vi "Execute.vi"(8 "error in (no error)":errorcluster, 9 "Workspace":T1, 10 "Control In":T2={"I-O.lvclass"=refnum, "Motion.lvclass"=refnum, "Dispenser.lvclass"=refnum}, 11 "Secure Syringe in":refnum<class "SecureRelease Syringe.lvclass">) -> (0 "error out":errorcluster, 2 "Control Out":T2, 3 "Secure Syringe out":refnum<class "SecureRelease Syringe.lvclass">)   [LabVIEW 2016, in "SecureRelease Syringe.lvclass"]
uses:
  SecureRelease Syringe.lvclass
  Controller/Controllers.ctl
  Controller/I-O/I-O.lvclass
  Controller/Motion/A3200/A3200.lvclass
  Controller/Dispenser/Dispenser.lvclass
  Controller/Motion/Motion.lvclass
  Workspace/Workspace.ctl
  SecureRelease Syringe.lvclass/SecureRelease Syringe.ctl
  Dispense/Dispense.lvclass
  Controller/Controller.lvclass
  Workspace/Fixture.lvclass
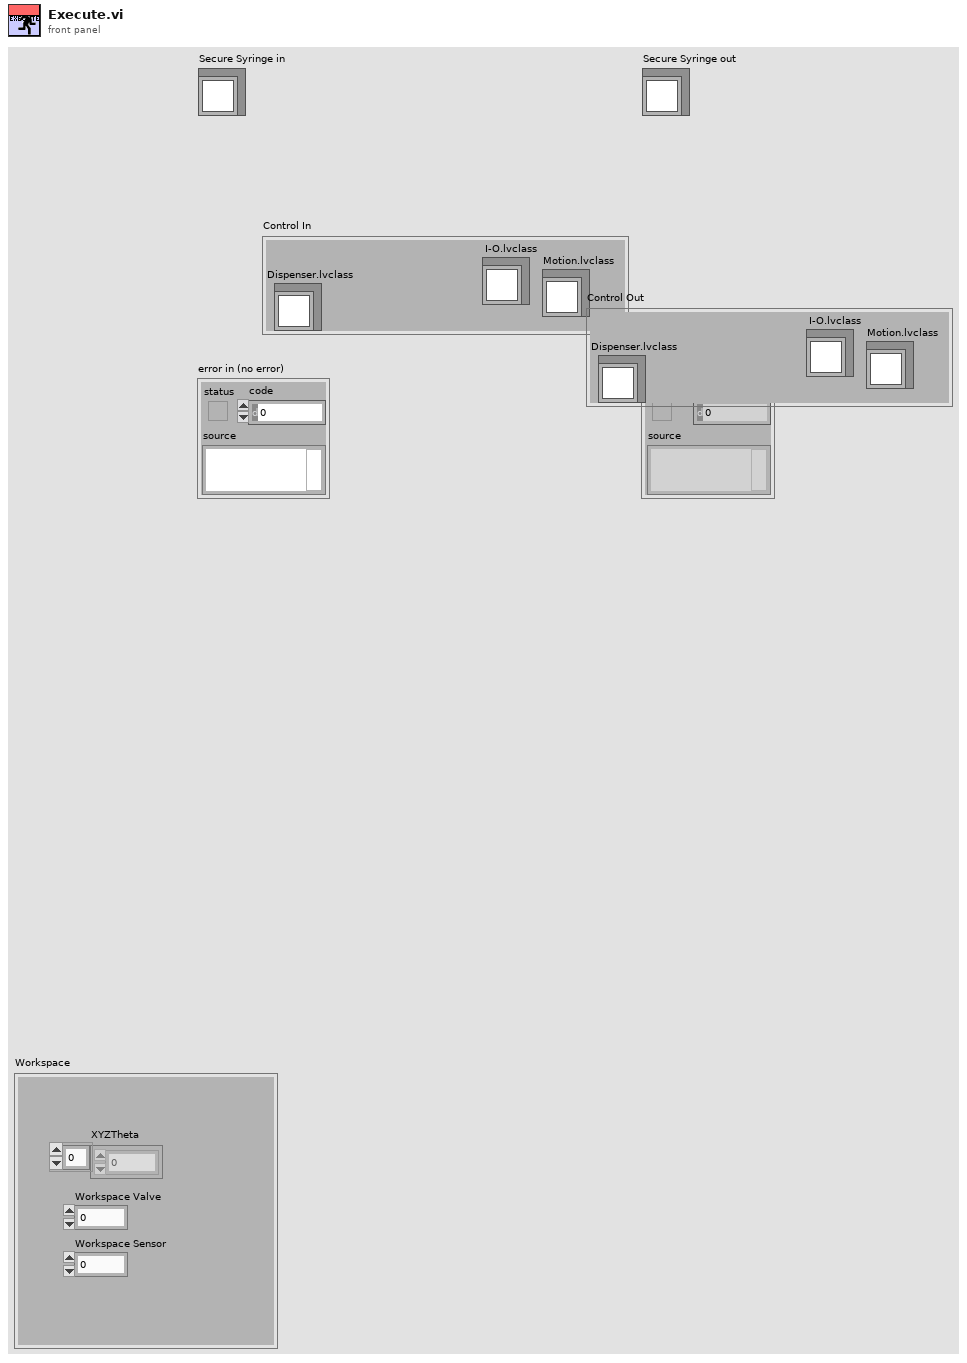
[diagram p1: front panel]
types:
  T1 = typedef "Fixture.lvclass/Workspace.ctl" = cluster{"XYZTheta":dbl[], "Workspace Valve":i32, "Workspace Sensor":i32}
  T2 = typedef "Controller.lvclass/Controllers.ctl" = cluster{"I-O.lvclass":refnum<class "I-O.lvclass">, "Motion.lvclass":refnum<class "Motion.lvclass">, "Dispenser.lvclass":refnum<class "Dispenser.lvclass">}
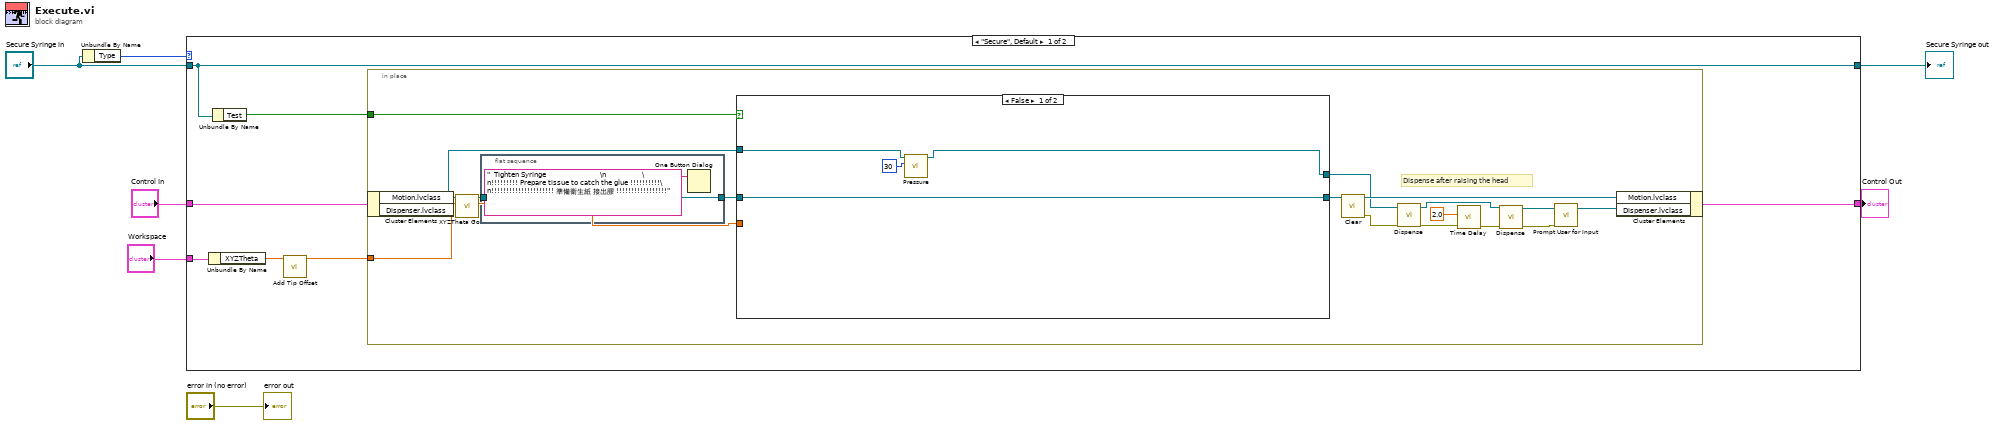
[diagram p0: block diagram]
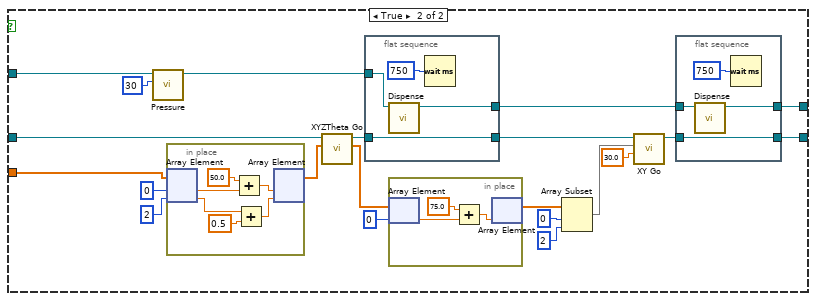
[diagram p2: hidden frame]
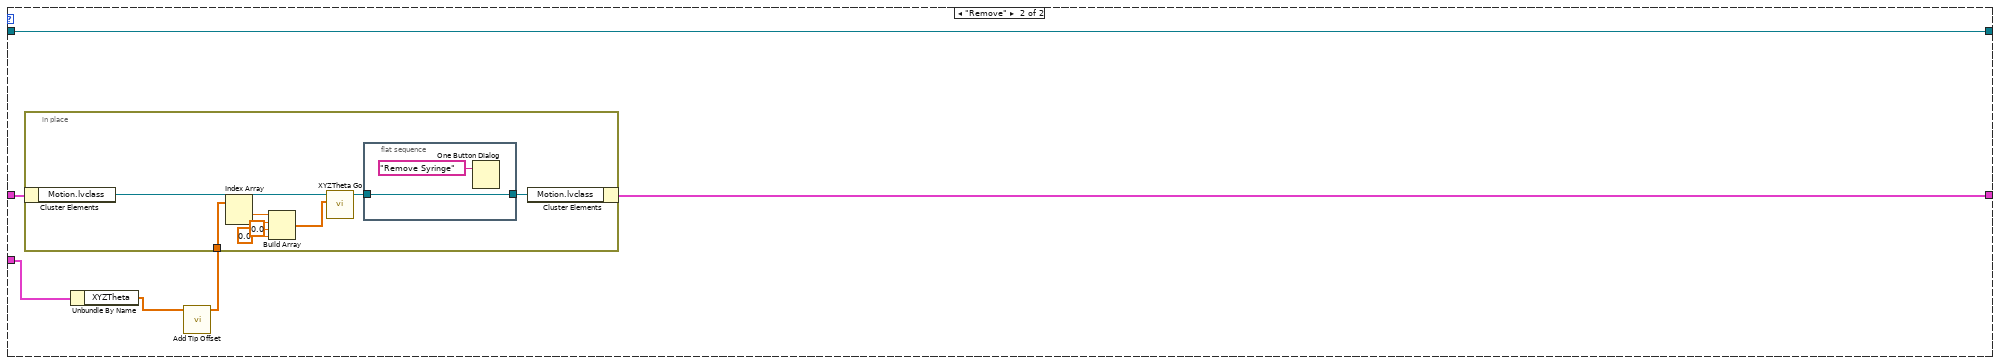
[diagram p3: hidden frame]
diagram:
  n1 = Unbundle By Name("Secure Syringe in") -> ("Type"=w1:enum16{"Secure", "Remove"})
  n2 = case shown="\"Secure\", Default" w1 {
    tunnel: "Workspace" -> [w14 w78]
    tunnel: "Secure Syringe in" -> [w10 w79]
    tunnel: [w10 w79] -> w5
    tunnel: "Control In" -> [w13 w80]
    tunnel: [w12 w81] -> w3
    frame "Secure", Default {
      n3 = Unbundle By Name(w14) -> ("XYZTheta"=w9:dbl[])
      n4 = Unbundle By Name(w10) -> ("Test"=w11:bool)
      n5 = call "Add Tip Offset.vi"("XYZTheta"=w9) -> ("XYZTheta"=w8:dbl[])  [unwired: 10 in]
      n6 = in-place {
        in-place-border: w8 -> [w30]
        in-place-border: w11 -> [w24]
        # "Dispense after raising the head"
        n7 = in-place-cluster #1(w13) -> ("Motion.lvclass"=w31:refnum<class "Motion.lvclass">, "Dispenser.lvclass"=w23:refnum<class "Dispenser.lvclass">)
        n8 = call "XYZTheta Go.vi"("XYZTheta In"=w30, "Motion in"=w31) -> ("XYZTheta Out"=w25:dbl[], "Motion out"=w29:refnum<class "Motion.lvclass">)  [unwired: 7 in, 1 out]
        n9 = flat-sequence {
          tunnel: [w32] -> w27
          tunnel: w29 -> [w32]
          frame #0 {
            n10 = One Button Dialog(message="  Tighten Syringe                           \n                  \n!!!!!!!!! Prepare tissue to catch the glue !!!!!!!!!!\n!!!!!!!!!!!!!!!!!!!!! 準備衛生紙 接出膠 !!!!!!!!!!!!!!!!!") -> ()  [unwired: 1 in, 1 out]
          }
        }
        n11 = case shown="False" w24 {
          tunnel: w27 -> [w37 w58]
          tunnel: [w37 w44] -> w26
          tunnel: w25 -> [_ w57]
          tunnel: w23 -> [w35 w50]
          tunnel: [w34 w42] -> w22
          frame False {
            n12 = call-dynamic "Pressure.vi"("Pressure"=i16 30, "Dispenser in"=w35) -> ("Dispenser out"=w34:refnum<class "Dispenser.lvclass">)  [unwired: 8 in, 1 out]
          }
          frame True {
            n13 = call-dynamic "Pressure.vi"("Pressure"=i16 30, "Dispenser in"=w50) -> ("Dispenser out"=w46:refnum<class "Dispenser.lvclass">)  [unwired: 8 in, 1 out]
            n14 = in-place {
              n15 = in-place-array #2(w57, 0, 2) -> (w75:dbl, w73:dbl)
              n16 = Add(x=50.0, y=w75) -> (x+y=w70:dbl)
              n17 = Add(x=w73, y=0.5) -> (x+y=w71:dbl)
              n18 = in-place-array #2(w70, w71) -> (w54:dbl[])  [unwired: 2 out]
            }
            n19 = call "XYZTheta Go.vi"("XYZTheta In"=w54, "Motion in"=w58) -> ("XYZTheta Out"=w53:dbl[], "Motion out"=w47:refnum<class "Motion.lvclass">)  [unwired: 7 in, 1 out]
            n20 = flat-sequence {
              tunnel: [w66] -> w48
              tunnel: w47 -> [w66]
              tunnel: w46 -> [w65]
              tunnel: [w63] -> w43
              frame #0 {
                n21 = call-dynamic "Dispense.vi"("Dispenser in"=w65) -> ("Dispenser out"=w63:refnum<class "Dispenser.lvclass">)  [unwired: 9 in, 1 out]
                n22 = Wait (ms)(milliseconds to wait=u32 750) -> ()  [unwired: 1 out]
              }
            }
            n23 = in-place {
              n24 = in-place-array #3(w53, 0) -> (w69:dbl)
              n25 = Add(x=75.0, y=w69) -> (x+y=w67:dbl)
              n26 = in-place-array #3(w67) -> (w41:dbl[])  [unwired: 1 out]
            }
            n27 = Array Subset(array=w41, index=0, length=2) -> (w38:dbl[])
            n28 = call-dynamic "XY Go.vi"("Speed"=30.0, "XY"=w38, "Motion in"=w48) -> ("Motion out"=w45:refnum<class "Motion.lvclass">)  [unwired: 7 in, 1 out]
            n29 = flat-sequence {
              tunnel: [w62] -> w44
              tunnel: w45 -> [w62]
              tunnel: w43 -> [w61]
              tunnel: [w59] -> w42
              frame #0 {
                n30 = call-dynamic "Dispense.vi"("Dispenser in"=w61) -> ("Dispenser out"=w59:refnum<class "Dispenser.lvclass">)  [unwired: 9 in, 1 out]
                n31 = Wait (ms)(milliseconds to wait=u32 750) -> ()  [unwired: 1 out]
              }
            }
          }
        }
        n32 = call "Clear.vi"("Motion in"=w26) -> ("error out"=w16:errorcluster, "Motion out"=w28:refnum<class "Motion.lvclass">)  [unwired: 9 in]
        n33 = call-dynamic "Dispense.vi"("error in (no error)"=w16, "Dispenser in"=w22) -> ("error out"=w21:errorcluster, "Dispenser out"=w20:refnum<class "Dispenser.lvclass">)  [unwired: 8 in]
        n34 = call "Time Delay"("error in (no error)"=w21, "Delay Time (s)"=2.0) -> ("error out"=w19:errorcluster)  [unwired: 9 in]
        n35 = call-dynamic "Dispense.vi"("error in (no error)"=w19, "Dispenser in"=w20) -> ("error out"=w15:errorcluster, "Dispenser out"=w18:refnum<class "Dispenser.lvclass">)  [unwired: 8 in]
        n36 = call "Prompt User for Input"("error in (no error)"=w15) -> ()  [unwired: 17 in, 2 out]
        n37 = in-place-cluster #1("Motion.lvclass"=w28, "Dispenser.lvclass"=w18) -> (w12:T2)
      }
    }
    frame "Remove" {
      n38 = Unbundle By Name(w78) -> ("XYZTheta"=w77:dbl[])
      n39 = call "Add Tip Offset.vi"("XYZTheta"=w77) -> ("XYZTheta"=w76:dbl[])  [unwired: 10 in]
      n40 = in-place {
        in-place-border: w76 -> [w87]
        n41 = in-place-cluster #4(w80) -> ("Motion.lvclass"=w90:refnum<class "Motion.lvclass">)
        n42 = Index Array(array=w87) -> (element #1=w86:dbl, element #2=w85:dbl)  [unwired: 2 in]
        n43 = Build Array(w86, w85, 0.0 ("element"), 0.0 ("element")) -> (w82:dbl[])
        n44 = call "XYZTheta Go.vi"("XYZTheta In"=w82, "Motion in"=w90) -> ("Motion out"=w89:refnum<class "Motion.lvclass">)  [unwired: 7 in, 2 out]
        n45 = flat-sequence {
          tunnel: w89 -> [w92]
          tunnel: [w92] -> w88
          frame #0 {
            n46 = One Button Dialog(message="Remove Syringe") -> ()  [unwired: 1 in, 1 out]
          }
        }
        n47 = in-place-cluster #4("Motion.lvclass"=w88) -> (w81:T2)
      }
    }
  }
  "Secure Syringe out" <- w5
  "Control Out" <- w3
  "error out" <- "error in (no error)"
